vi "Tag_Buffer_Dbl_PID_VIG.vi"(7 "Operation":T1(ring)=enum."set all data", 8 "error in":errorcluster, 11 "tag_data_in":dbl[](array[numeric])) -> (0 "error out":errorcluster, 3 "tag_data_out":dbl[](array[numeric]))   [LabVIEW 2018]
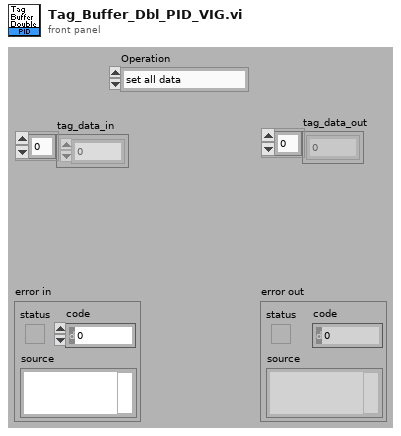
[diagram p1: front panel]
types:
  T1 = enum16{"get data", "set all data", "set Process Variable", "initialize"}
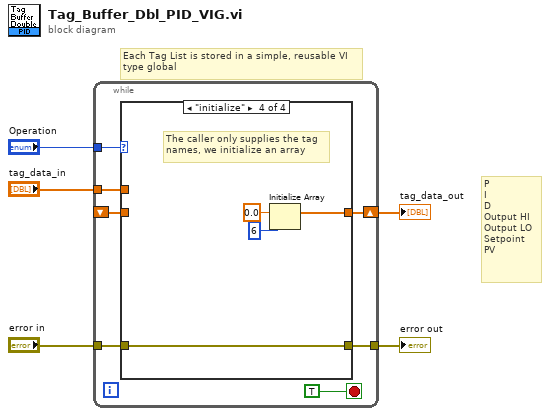
[diagram p0: block diagram]
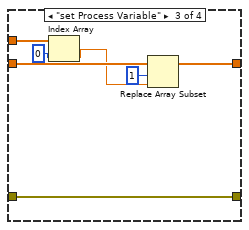
[diagram p4: hidden frame]
diagram:
  # "P\nI\nD\nOutput HI\nOutput LO\nSetpoint\nPV"
  # "Each Tag List is stored in a simple, reusable VI\ntype global"
  n1 = while {
    tunnel: "Operation" -> [w12]
    shift-right: [w10] -> w3
    shift-left: _ -> [w8]
    tunnel: "tag_data_in" -> [w9]
    tunnel: "error in" -> [w7]
    tunnel: [w6] -> w1
    stop <- TRUE stop-if-true
    n2 = case shown="\"initialize\"" w12 {
      tunnel: [w14 w16 w18 w27] -> w10
      tunnel: w9 -> [_ w16 w22 _]
      tunnel: w8 -> [w14 _ w20 _]
      tunnel: w7 -> [w13 w15 w23 w26]
      tunnel: [w13 w15 w23 w26] -> w6
      frame "get data", Default {
      }
      frame "set all data" {
        # "For speed, we only set the\ndata, not the tag names."
      }
      frame "set Process Variable" {
        n3 = Index Array(array=w22, index=0) -> (element=w17:dbl)
        n4 = Replace Array Subset(array=w20, new element=w17, index=1) -> (w18:dbl[])
      }
      frame "initialize" {
        # "The caller only supplies the tag\nnames, we initialize an array"
        n5 = Initialize Array(0.0 ("element"), 6 ("dimension size")) -> (w27:dbl[])
      }
    }
  }
  "error out" <- w1
  "tag_data_out" <- w3
